vi "LM35_ARDUNIO_labview_rx_tx.vi"() -> ()   [LabVIEW 2014]
uses:
  <vilib>/Instr/_visa.llb/VISA Configure Serial Port (Instr).vi
panel:
  in  "stop bits (10: 1 bit)":u16(ring)=10 items=["1.0"=10, "1.5"=15, "2.0"=20]
  in  "parity (0:none)":enum16{"None", "Odd", "Even", "Mark", "Space"}(ring)
  in  "data bits (8)":u16=8 min=5 max=8 step=1
  in  "baud rate (9600)":u32=9600
  out "TEMPERATURE in 0C":dbl(slide) scale=0.0..100.0
  in  "stop":bool
  out "TEMP. WAVFORM":i32(graph)
  out "TEMPERATURE in 0C":string
  out "SERIAL DATA BUFFER":string
  in  "byte count":u32
  in  "VISA resource name":refnum<visa-resource-name>
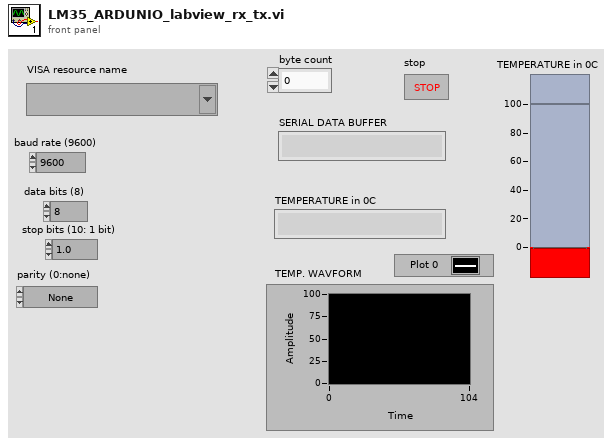
[diagram p1: front panel]
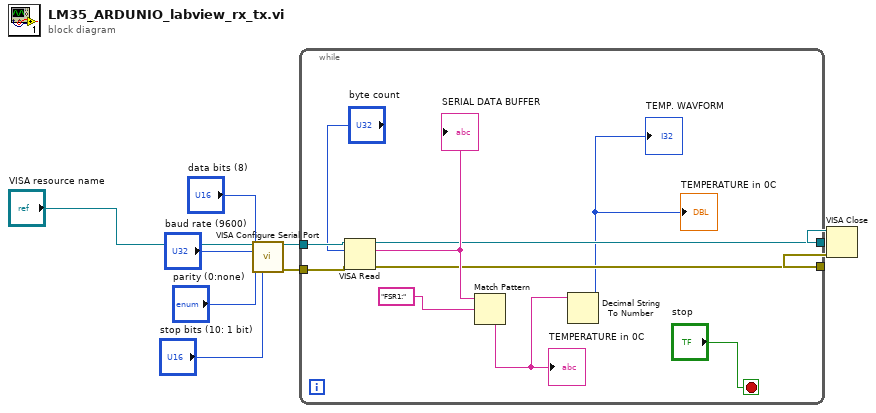
[diagram p0: block diagram]
diagram:
  n1 = call-poly "VISA Configure Serial Port"("VISA resource name"="VISA resource name", "baud rate (9600)"="baud rate (9600)", "data bits (8)"="data bits (8)", "parity (0:none)"="parity (0:none)", "stop bits (10: 1 bit)"="stop bits (10: 1 bit)") -> ("VISA resource name out"=w8:refnum<visa-resource-name>, "error out"=w7:errorcluster)  [unwired: 9 in]
  n2 = while {
    tunnel: w8 -> [w19]
    tunnel: w7 -> [w18]
    tunnel: [w13] -> w6
    tunnel: [w12] -> w5
    stop <- "stop" stop-if-true
    n3 = VISA Read(VISA resource name=w19, byte count="byte count", error in (no error)=w18) -> (VISA resource name out=w12:refnum<visa-resource-name>, read buffer=w16:string, error out=w13:errorcluster)  [unwired: 1 out]
    "SERIAL DATA BUFFER" <- w16
    n4 = Match Pattern(string=w16, regular expression="FSR1:") -> (after substring=w14:string)  [unwired: 1 in, 3 out]
    "TEMPERATURE in 0C" <- w14
    n5 = Decimal String To Number(string=w14) -> (number=→"TEMP. WAVFORM" →"TEMPERATURE in 0C":i32)  [unwired: 2 in, 1 out]
  }
  n6 = VISA Close(VISA resource name=w5, error in (no error)=w6) -> ()  [unwired: 1 out]
